vi "Configure Individual Limit Test.vi"(0 "VISA resource name":refnum<visa-resource-name>, 1 "Enable Limit Test (F: Disable)":bool, 2 "Limit Test Upper Limit (1)":dbl=1.0, 5 "Channel (1: Channel 1)":i32(ring)=1 items=["Channel 1"=1, "Channel 2"=2], 7 "Limit Test Number (1)":i32=1, 9 "Limit Test Type (1: Limit)":i32(ring)=1 items=["Compliance", "Limit"], 11 "error in (no error)":errorcluster, 12 "Compliance Test Judgement Criteria (1: Out)":i32(ring)=1 items=["In", "Out"], 13 "Limit Test Lower Limit (-1)":dbl=-1.0) -> (4 "VISA resource name out":refnum<visa-resource-name>, 15 "error out":errorcluster)   [LabVIEW 2012, in "Keysight B2980 Series.lvlib"]
doc: "Configures the properties of specified limit test. . The limit test is a pass/fail judgment performed during a composite limit test. The limit test result is returned by ReadLimitTestResult."
uses:
  Keysight B2980 Series.lvlib
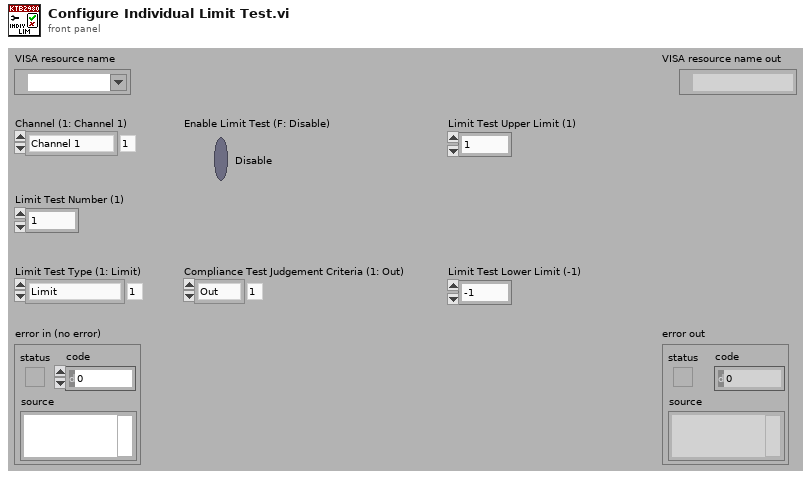
[diagram p1: front panel]
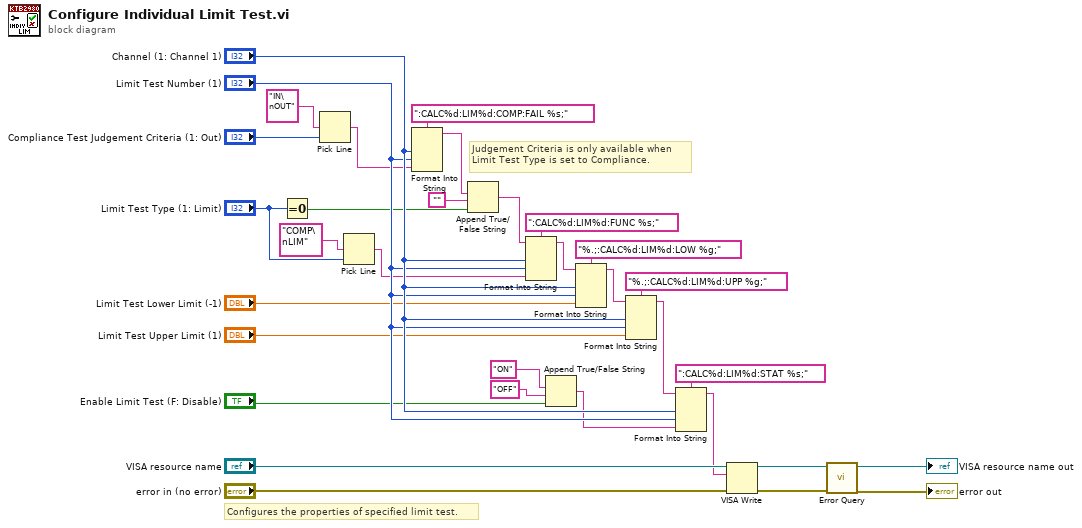
[diagram p0: block diagram]
diagram:
  # "Judgement Criteria is only available when\nLimit Test Type is set to Compliance."
  # "Configures the properties of specified limit test."
  n1 = Equal To 0?(x="Limit Test Type (1: Limit)") -> (x = 0?=w5:bool)
  n2 = Pick Line(multi-line string="IN\nOUT", line index="Compliance Test Judgement Criteria (1: Out)") -> (output string=w28:string)  [unwired: 1 out]
  n3 = Pick Line(multi-line string="COMP\nLIM", line index="Limit Test Type (1: Limit)") -> (output string=w25:string)  [unwired: 1 out]
  n4 = Format Into String(format string=":CALC%d:LIM%d:COMP:FAIL %s;", "Channel (1: Channel 1)", "Limit Test Number (1)", w28) -> (resulting string=w4:string)  [unwired: 2 in, 1 out]
  n5 = Append True/False String(1:w5, 2:"", 3:w4) -> (0:w2:string)  [unwired: 1 out]
  n6 = Format Into String(format string=":CALC%d:LIM%d:FUNC %s;", initial string=w2, "Channel (1: Channel 1)", "Limit Test Number (1)", w25) -> (resulting string=w24:string)  [unwired: 1 in, 1 out]
  n7 = Append True/False String(1:"Enable Limit Test (F: Disable)", 2:"OFF", 3:"ON") -> (0:w13:string)  [unwired: 1 out]
  n8 = Format Into String(format string="%.;:CALC%d:LIM%d:LOW %g;", initial string=w24, "Channel (1: Channel 1)", "Limit Test Number (1)", "Limit Test Lower Limit (-1)") -> (resulting string=w21:string)  [unwired: 1 in, 1 out]
  n9 = Format Into String(format string="%.;:CALC%d:LIM%d:UPP %g;", initial string=w21, "Channel (1: Channel 1)", "Limit Test Number (1)", "Limit Test Upper Limit (1)") -> (resulting string=w15:string)  [unwired: 1 in, 1 out]
  n10 = Format Into String(format string=":CALC%d:LIM%d:STAT %s;", initial string=w15, "Channel (1: Channel 1)", "Limit Test Number (1)", w13) -> (resulting string=w1:string)  [unwired: 1 in, 1 out]
  n11 = VISA Write(VISA resource name="VISA resource name", write buffer=w1, error in (no error)="error in (no error)") -> (VISA resource name out=w10:refnum<visa-resource-name>, error out=w9:errorcluster)  [unwired: 1 out]
  n12 = call "Error Query.vi"("error in (no error)"=w9, "VISA resource name"=w10) -> ("error out"=→"error out":errorcluster, "VISA resource name out"=→"VISA resource name out":refnum<visa-resource-name>)  [unwired: 8 out]
